vi "AutoDriveStraightWeird.vi"(8 "error in (no error)":errorcluster, 9 "TimeOut (s)":dbl, 10 "MaxSpeed (ft/s)":dbl, 11 "Dist (ft)":dbl) -> (0 "error out":errorcluster)   [LabVIEW 2020]
doc: "Wrapper class for drive straight"
uses:
  <vilib>/Rock Robotics/WPI/ThirdParty/JAS_Junk/TrajLib/Trajectory_Library.lvlib
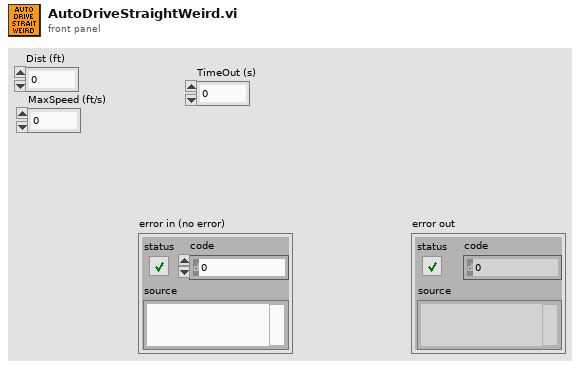
[diagram p1: front panel]
types:
  T1 = typedef "Trajectory_Library.lvlib/TIMER.ctl" = cluster{"StartTime":dbl, "Accumulated TIme":dbl, "Running":bool, "semaphore":T2}
  T2 = typedef "Semaphore RefNum" = refnum<k1>
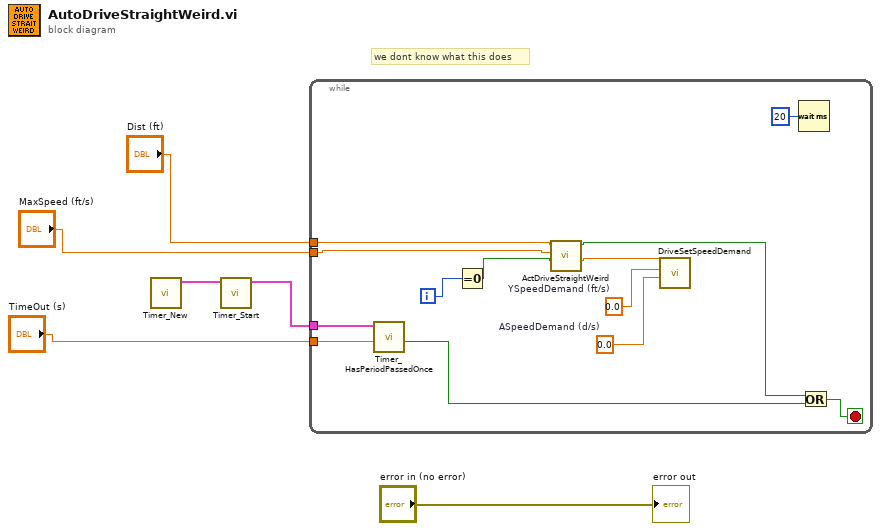
[diagram p0: block diagram]
diagram:
  # "we dont know what this does"
  n1 = call <vilib>:"Timer_New.vi"() -> ("TIMER"=w3:T1)  [unwired: 11 in]
  n2 = call <vilib>:"Timer_Start.vi"("in Timer"=w3) -> ("out Timer"=w2:T1)  [unwired: 10 in]
  n3 = while {
    tunnel: "Dist (ft)" -> [w9]
    tunnel: "MaxSpeed (ft/s)" -> [w10]
    tunnel: w2 -> [w18]
    tunnel: "TimeOut (s)" -> [w17]
    i -> [w19]
    stop <- w15 stop-if-true
    w7 = 0.0  # YSpeedDemand (ft/s)
    w8 = 0.0  # ASpeedDemand (d/s)
    n4 = call <vilib>:"Timer_HasPeriodPassedOnce.vi"("Period"=w17, "in Timer"=w18) -> ("Expired"=w16:bool)  [unwired: 7 in, 2 out]
    n5 = Equal To 0?(x=w19) -> (x = 0?=w11:bool)
    n6 = call "ActDriveStraightWeird.vi"("FirstTime"=w11, "MaxSpeed (ft/s)"=w10, "Dist (ft)"=w9) -> ("LeftSpeedDemand"=w13:dbl, "Done"=w12:bool)  [unwired: 6 in, 1 out]
    n7 = call "DriveSetSpeedDemand.vi"("ASpeedDemand (d/s)"=w8, "YSpeedDemand (ft/s)"=w7, "XSpeedDemand (ft/s)"=w13) -> ()  [unwired: 9 in]
    n8 = Wait (ms)(milliseconds to wait=u32 20) -> ()  [unwired: 1 out]
    n9 = Or(x=w12, y=w16) -> (x .or. y?=w15:bool)
  }
  "error out" <- "error in (no error)"
